vi "Random Number.vi"(0 "Maximum":dbl=500.0, 1 "Minimum":dbl=100.0) -> (6 "Integer":i64, 7 "Double":dbl, 8 "?":string)   [LabVIEW 2020]
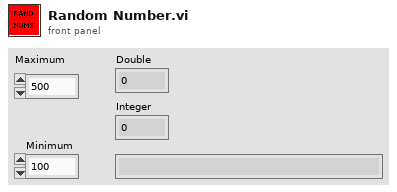
[diagram p1: front panel]
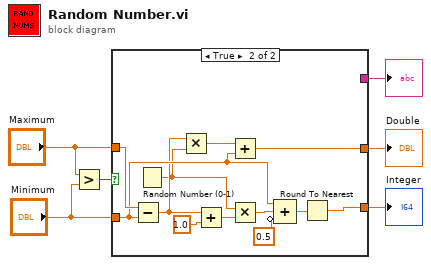
[diagram p0: block diagram]
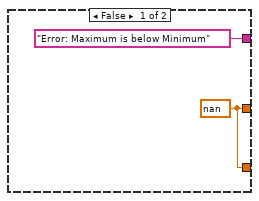
[diagram p2: hidden frame]
diagram:
  n1 = Greater?(x="Maximum", y="Minimum") -> (0:w6:bool)
  n2 = case shown="True" w6 {
    tunnel: "Maximum" -> [_ w20]
    tunnel: "Minimum" -> [_ w14]
    tunnel: [w7 w18] -> w3
    tunnel: ["Error: Maximum is below Minimum" _] -> w2
    tunnel: [w7 w17] -> w1
    frame False {
      w7 = nan
    }
    frame True {
      n3 = Subtract(x=w20, y=w14) -> (x-y=w13:dbl)
      n4 = Random Number (0-1)() -> (number: 0 to 1=w11:dbl)
      n5 = Multiply(x=w13, y=w11) -> (x*y=w19:dbl)
      n6 = Add(x=w13, y=1.0) -> (x+y=w12:dbl)
      n7 = Add(x=w19, y=w14) -> (x+y=w18:dbl)
      n8 = Multiply(x=w11, y=w12) -> (x*y=w15:dbl)
      n9 = Compound Arithmetic op=ADD(w14, w15, invert 0.5 ("value")) -> (w16:dbl)
      n10 = Round To Nearest(number=w16) -> (nearest integer value=w17:dbl)
    }
  }
  "Double" <- w3
  "?" <- w2
  "Integer" <- w1
